vi "onGenerateNewInboundChannel.vi"(8 "error in (no error)":errorcluster, 11 "Connection.TCP in":refnum<class "Connection.TCP.lvclass">) -> (0 "error out":errorcluster, 3 "Connection.TCP out":refnum<class "Connection.TCP.lvclass">)   [LabVIEW 2013, in "Connection.TCP_GOSPL.lvlib" / "Connection.TCP.lvclass"]
uses:
  Connection.TCP.lvclass
  Connection/Connection.lvclass
  Connection/Connection.lvclass/Connection.ctl
  Connection.TCP.lvclass/Connection.TCP.ctl
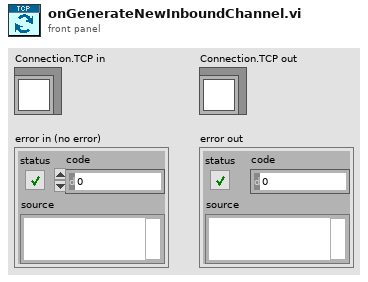
[diagram p1: front panel]
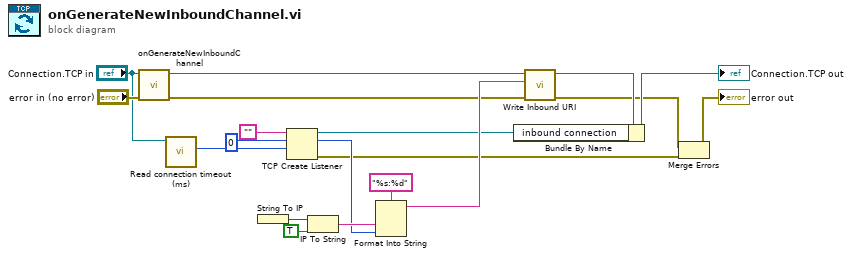
[diagram p0: block diagram]
diagram:
  n1 = call-parent "onGenerateNewInboundChannel.vi"("error in (no error)"="error in (no error)", "Connection in"="Connection.TCP in") -> ("error out"=w2:errorcluster, "Connection out"=w17:refnum<class "Connection.TCP.lvclass">)  [unwired: 8 in]
  n2 = call "Read connection timeout (ms).vi"("Connection in"="Connection.TCP in") -> ("connection timeout (ms)"=w9:i32)  [unwired: 8 in, 2 out]
  n3 = String To IP() -> (0:w8:u32)  [unwired: 1 in]
  n4 = TCP Create Listener(9:w9, 10:u16 0 ("port"), 11:"") -> (0:w3:errorcluster, 2:w4:u16, 3:w13:refnum<k5>)  [unwired: 2 in]
  n5 = IP To String(1:TRUE ("dot notation? (F)"), 2:w8) -> (0:w6:string)
  n6 = Format Into String(format string="%s:%d", w6, w4) -> (resulting string=w14:string)  [unwired: 2 in, 1 out]
  n7 = call "Write Inbound URI.vi"("Inbound URI"=w14, "Connection in"=w17) -> ("Connection out"=w12:refnum<class "Connection.TCP.lvclass">)  [unwired: 9 in]
  n8 = Bundle By Name(cluster=w12, "inbound connection"=w13) -> (→"Connection.TCP out":refnum<class "Connection.TCP.lvclass">)
  n9 = Merge Errors(w2, w3) -> (→"error out":errorcluster)
